vi "sync_with_globals.vi"(4 "Selection/Group":T3[](array[typedef]), 7 "Spots":T1[](array[typedef]) {"Amplitude Correction" step=0.1; "Line Trapping"."Phase Gradient" step=0.05; "Line Trapping"."Vector"."x" step=1e-06 format="%#_6p"; "Line Trapping"."Vector"."y" step=1e-06 format="%#_6p"; "Line Trapping"."Vector"."z" step=1e-06 format="%#_6p"; "NA Position"."r" step=1e-06; "NA Position"."y" step=1e-06; "NA Position"."x" step=1e-06; "Position"."z" step=1e-06; "Position"."y" step=1e-06; "Position"."x" step=1e-06; "Phase" step=0.7753; "Intensity" step=0.1}) -> (0 "Selection/Group 2":T3[](array[typedef]), 3 "Spots 2":T1[](array[typedef]) {"Amplitude Correction" step=0.1; "Line Trapping"."Phase Gradient" step=0.05; "Line Trapping"."Vector"."x" step=1e-06 format="%#_6p"; "Line Trapping"."Vector"."y" step=1e-06 format="%#_6p"; "Line Trapping"."Vector"."z" step=1e-06 format="%#_6p"; "NA Position"."r" step=1e-06; "NA Position"."y" step=1e-06; "NA Position"."x" step=1e-06; "Position"."z" step=1e-06; "Position"."y" step=1e-06; "Position"."x" step=1e-06; "Phase" step=0.7753; "Intensity" step=0.1})   [LabVIEW 2015]
doc: "Sync spots with global variables: if the spots have changed since the last time this VI was run, it updates the global variables. Otherwise, it replaces the spots we currently have with the contents of the global variables. This allows \"remote control\" of this program by other programs, including plugins."
uses:
  selection_element.ctl
  spot.ctl
  line_trapping.ctl
  red_tweezers_globals.vi
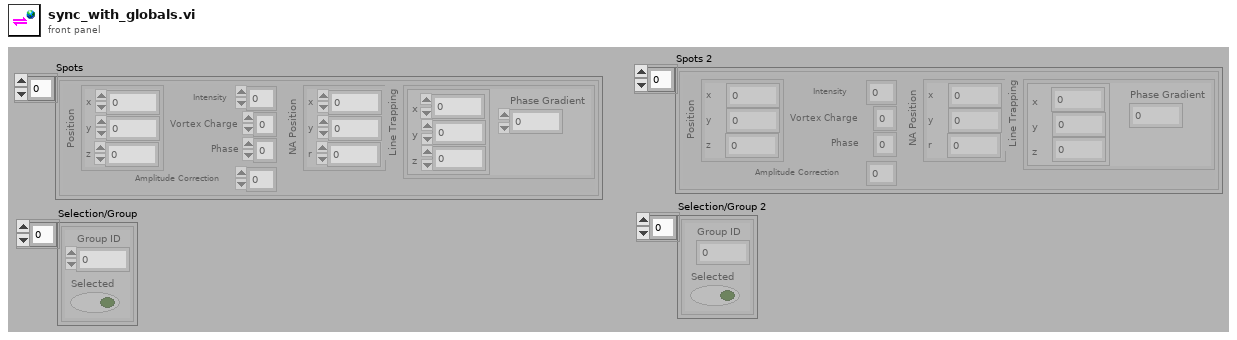
[diagram p1: front panel]
types:
  T1 = typedef "spot.ctl" = cluster{"Position":cluster{"x":dbl, "y":dbl, "z":dbl}, "Intensity":dbl, "Vortex Charge":i8, "Phase":dbl, "NA Position":cluster{"x":dbl, "y":dbl, "r":dbl}, "Line Trapping":T2, "Amplitude Correction":dbl}
  T2 = typedef "line_trapping.ctl" = cluster{"Vector":cluster{"x":dbl, "y":dbl, "z":dbl}, "Phase Gradient":dbl}
  T3 = typedef "selection_element.ctl" = cluster{"Group ID":i32, "Selected":bool}
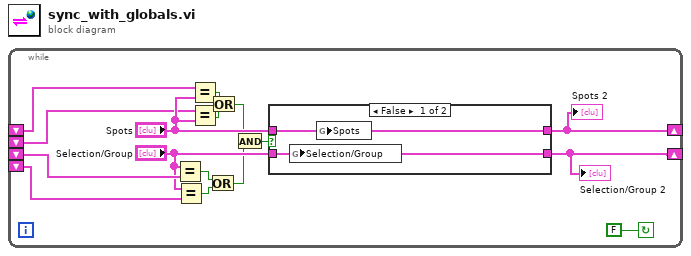
[diagram p0: block diagram]
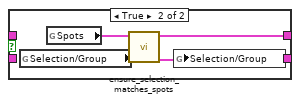
[diagram p2: hidden frame]
diagram:
  n1 = while {
    shift-right: [w14] -> _
    shift-left: _ -> [w13]
    shift-right: [w15] -> _
    shift-left: _ -> [w12]
    shift-left: _ -> [w10]
    shift-left: _ -> [w5]
    stop <- FALSE continue-if-true
    n2 = Equal?(x="Selection/Group", y=w12) -> (x = y?=w2:bool)
    n3 = Equal?(x="Selection/Group", y=w5) -> (x = y?=w3:bool)
    n4 = Equal?(x=w13, y="Spots") -> (x = y?=w7:bool)
    n5 = Equal?(x=w10, y="Spots") -> (x = y?=w8:bool)
    n6 = Or(x=w2, y=w3) -> (x .or. y?=w1:bool)
    n7 = Or(x=w7, y=w8) -> (x .or. y?=w9:bool)
    n8 = And(x=w9, y=w1) -> (x .and. y?=w6:bool)
    n9 = case shown="False" w6 {
      tunnel: [w17 w22] -> w14
      tunnel: "Spots" -> [w17 _]
      tunnel: "Selection/Group" -> [w18 _]
      tunnel: [w18 w19] -> w15
      frame False {
        n10 = global write "red_tweezers_globals.vi" "Selection/Group"(w18) -> ()
        n11 = global write "red_tweezers_globals.vi" "Spots"(w17) -> ()
      }
      frame True {
        n12 = global read "red_tweezers_globals.vi" "Selection/Group"() -> (w21:T3[])
        n13 = global read "red_tweezers_globals.vi" "Spots"() -> (w20:T1[])
        n14 = call "ensure_selection_matches_spots.vi"("Selection and Groups in"=w21, "Spots"=w20) -> ("Selection and Groups out"=w19:T3[], "Spots (duplicate)"=w22:T1[])  [unwired: 4 in]
        n15 = global write "red_tweezers_globals.vi" "Selection/Group"(w19) -> ()
      }
    }
    "Selection/Group 2" <- w15
    "Spots 2" <- w14
  }
